vi "Inversor tensões.vi"(3 "In 2":dbl, 4 "In 1":dbl, 5 "Dados":dbl[](array[numeric])) -> (0 "Out 2":dbl, 1 "Out 1":dbl)   [LabVIEW 2018]
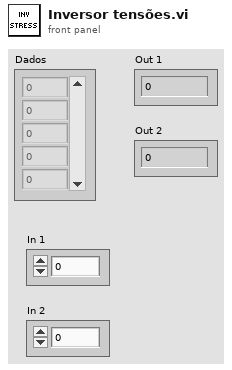
[diagram p1: front panel]
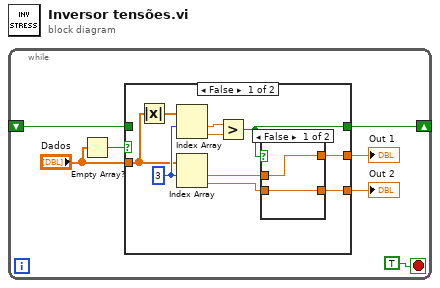
[diagram p0: block diagram]
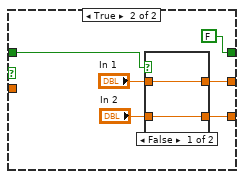
[diagram p3: hidden frame]
diagram:
  n1 = while {
    shift-right: [w2] -> _
    shift-left: _ -> [w1]
    stop <- TRUE stop-if-true
    n2 = Empty Array?(array="Dados") -> (empty?=w3:bool)
    n3 = case shown="False" w3 {
      tunnel: "Dados" -> [w11 _]
      tunnel: [w14 w24] -> w5
      tunnel: [w13 w22] -> w6
      tunnel: [w8 FALSE] -> w2
      tunnel: w1 -> [_ w26]
      frame False {
        w12 = 3 ("index")
        n4 = Absolute Value(x=w11) -> (abs(x)=w15:dbl[])
        n5 = Index Array(array=w15, index #1=w12) -> (element #1=w17:dbl, element #2=w16:dbl)  [unwired: 1 in]
        n6 = Index Array(array=w11, index #1=w12) -> (element #1=w10:dbl, element #2=w9:dbl)  [unwired: 1 in]
        n7 = Greater?(x=w17, y=w16) -> (0:w8:bool)
        n8 = case shown="False" w8 {
          tunnel: [w18 w21] -> w14
          tunnel: w10 -> [w19 w21]
          tunnel: w9 -> [w18 w20]
          tunnel: [w19 w20] -> w13
          frame False {
          }
          frame True {
          }
        }
      }
      frame True {
        n9 = case shown="False" w26 {
          tunnel: "In 1" -> [w29 w31]
          tunnel: [w28 w31] -> w24
          tunnel: "In 2" -> [w28 w30]
          tunnel: [w29 w30] -> w22
          frame False {
          }
          frame True {
          }
        }
      }
    }
    "Out 1" <- w6
    "Out 2" <- w5
  }
